vi "divide.vi"(1 "c":bool, 2 "INPUT":T2) -> (0 "OUTPUT":T1)   [LabVIEW 2013]
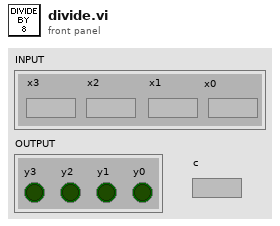
[diagram p1: front panel]
types:
  T1 = cluster{"y3":bool, "y2":bool, "y1":bool, "y0":bool}
  T2 = cluster{"x0":bool, "x1":bool, "x2":bool, "x3":bool}
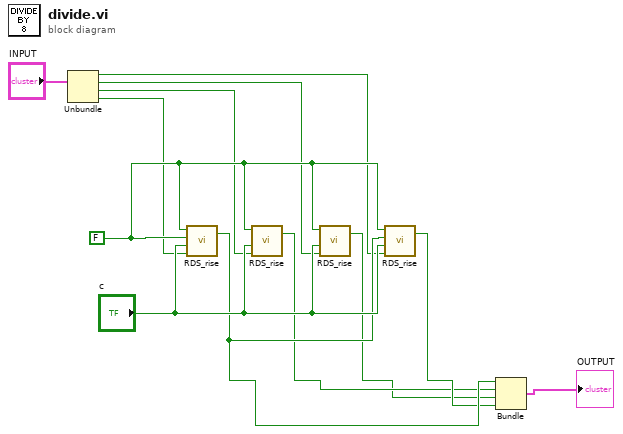
[diagram p0: block diagram]
diagram:
  w11 = FALSE
  n1 = Unbundle("INPUT") -> ("x0"=w4:bool, "x1"=w3:bool, "x2"=w2:bool, "x3"=w1:bool)
  n2 = call "RDS_rise.vi"("S"=w1, "C"="c", "D"=w11, "R"=w11) -> ("Q"=w10:bool)  [unwired: 1 out]
  n3 = call "RDS_rise.vi"("S"=w2, "C"="c", "R"=w11) -> ("Q"=w8:bool)  [unwired: 1 in, 1 out]
  n4 = call "RDS_rise.vi"("S"=w3, "C"="c", "R"=w11) -> ("Q"=w7:bool)  [unwired: 1 in, 1 out]
  n5 = call "RDS_rise.vi"("S"=w4, "C"="c", "D"=w10, "R"=w11) -> ("Q"=w9:bool)  [unwired: 1 out]
  n6 = Bundle("Q"=w10, "Q"=w8, "Q"=w7, "Q"=w9) -> (→"OUTPUT":cluster{"Q":bool, "Q":bool, "Q":bool, "Q":bool})  [unwired: 1 in]
